vi "Vision Research Phantom Series PhCon PhNVMSave.vi"(0 "CN in":u32=1, 1 "Cine":i32, 5 "Error In (no error)":errorcluster, 7 "CallID":u32) -> (14 "CN out":u32=1, 19 "Error Out":errorcluster)   [LabVIEW 2013, in "VRI.lvlib"]
doc: "PhCon.dll\n\nPhNVMSave\nHRESULT PhNVMSave(UINT CN, int Cine, UINT CallID);\n\nParameters Description\nCN (in) Camera number\nCineNo (in) Cine number\nCallID (in) Choose a CallID(unsigned int <= 15) and pass it \n in the place of the Function pointer parameter.\n To retrieve progress information for that call, \n you must call LVProgress with chosen CallID \n within a loop.\n The time consuming call and the LVProgress call \n must be in separate threads.\nReturn HRESULT (0=Ok)\nComments Save the cine recorded in DRAM to the \n NonVolatile memory (to the next free position)\n\nWritten by:\nBLOOMY CONTROLS, INC\nWINDSOR, CT 06095, USA\n860-298-9925\nwww.bloomy.com\nV1.0.0\nMay, 2004hicð.0\nMay,"
uses:
  VRI.lvlib
  Phantom DLLs/PhCon.Dll
panel:
  # "For instructions on the use of this VI, press Ctrl+H to display the help window and move the mouse over the icon, controls, and indicators"
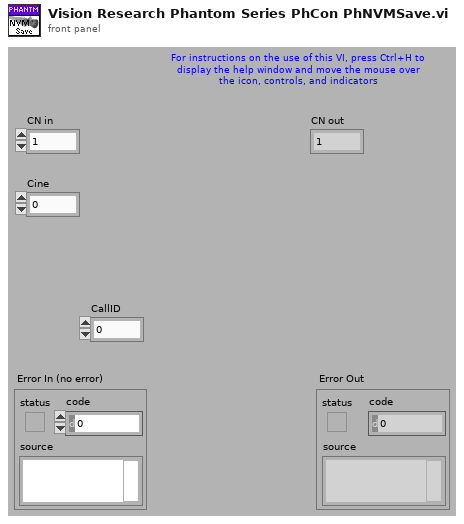
[diagram p1: front panel]
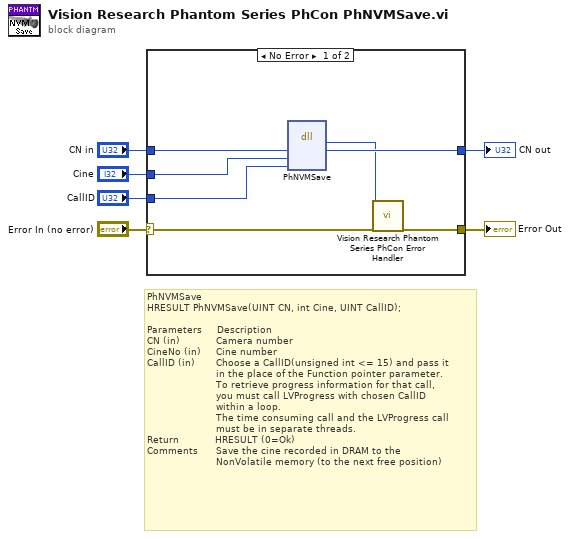
[diagram p0: block diagram]
diagram:
  # "PhNVMSave\nHRESULT PhNVMSave(UINT CN, int Cine, UINT CallID);\n\nParameters     Description\nCN (in)            Camera number\nCineNo (in)     Cine number\nCallID (in)       Choose a CallID(unsigned int <= 15) and pass it \n                       in the place of the Function pointer parameter.\n                       To retrieve progress information for that call, \n                       you must call LVProgress with chosen CallID \n                       within a loop.\n                       The time consuming call and the LVProgress call \n                       must be in separate threads.\nReturn            HRESULT (0=Ok)\nComments      Save the cine recorded in DRAM to the \n                       NonVolatile memory (to the next free position)"
  n1 = case shown="No Error" "Error In (no error)" {
    selector: "Error In (no error)" -> [w13 w15]
    tunnel: [w12 w15] -> w5
    tunnel: "CN in" -> [w11 w14]
    tunnel: [w10 w14] -> w3
    tunnel: "Cine" -> [w9 _]
    tunnel: "CallID" -> [w8 _]
    frame No Error {
      n2 = dll-call lib="C:/Projects/SDK/64-bit/Vision Research Phantom Series Labview Driver/Phantom DLLs/PhCon.dll" fn="PhNVMSave"("CN"=w11, "Cine"=w9, "CallID"=w8) -> ("HRESULT"=w7:i32, "CN"=w10:u32)  [unwired: 5 in, 2 out]
      n3 = call "Vision Research Phantom Series PhCon Error Handler.vi"("ErrNo"=w7, "Error In (no error)"=w13) -> ("Error Out"=w12:errorcluster)  [unwired: 17 out]
    }
    frame Error {
    }
  }
  "Error Out" <- w5
  "CN out" <- w3
